vi "Select DB.vi"(8 "error in (no error)":errorcluster, 10 "DB Type":T1, 11 "Sim Configuration Database Actor in":refnum<class "Sim Configuration Database Actor.lvclass">) -> (0 "error out":errorcluster, 3 "Sim Configuration Database Actor out":refnum<class "Sim Configuration Database Actor.lvclass">)   [LabVIEW 2019, in "Sim Configuration Database Actor.lvlib" / "Sim Configuration Database Actor.lvclass"]
uses:
  Sim Configuration Database Actor.lvclass
  Database Type.ctl
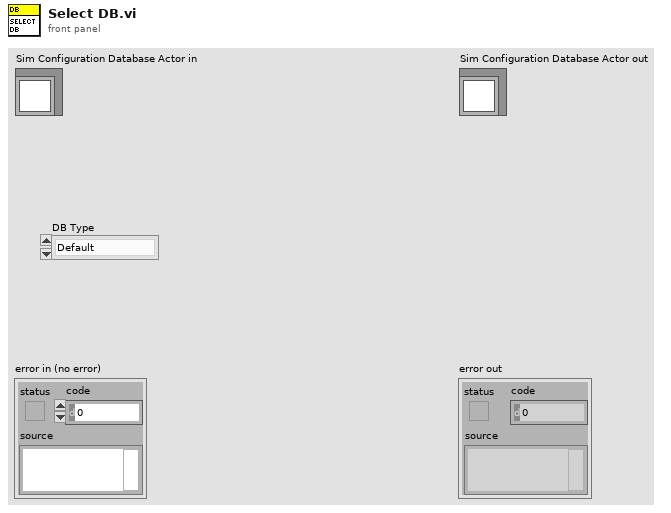
[diagram p1: front panel]
types:
  T1 = typedef "Sim Configuration Database Actor.lvlib/Sim Configuration Database Actor.lvclass/Database Type.ctl" = enum16{"Default", "Client"}
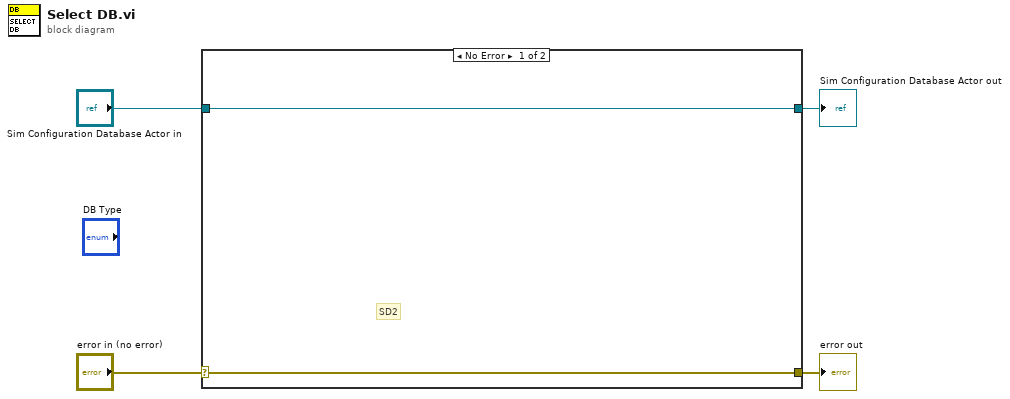
[diagram p0: block diagram]
diagram:
  n1 = case shown="No Error" "error in (no error)" {
    selector: "error in (no error)" -> [w5 w8]
    tunnel: [w5 w8] -> w3
    tunnel: [w6 w7] -> w1
    tunnel: "Sim Configuration Database Actor in" -> [w6 w7]
    frame No Error {
      # "SD2"
    }
    frame Error {
    }
  }
  "error out" <- w3
  "Sim Configuration Database Actor out" <- w1
